vi "Write Roles.vi"(8 "error in (no error)":errorcluster, 10 "Roles":T1, 11 "NormalGamePlay in":refnum<class "NormalGamePlay.lvclass">) -> (0 "error out":errorcluster, 3 "NormalGamePlay out":refnum<class "NormalGamePlay.lvclass">)   [LabVIEW 2020, in "NormalGamePlay.lvclass"]
uses:
  NormalGamePlay.lvclass
  ShootRole_class/ShootRole.lvclass
  FollowAttackerRole_class/FollowAttackerRole.lvclass
  DefaultPsRole_class/DefaultPsRole.lvclass
  NormalGamePlay.lvclass/NormalGamePlay.ctl
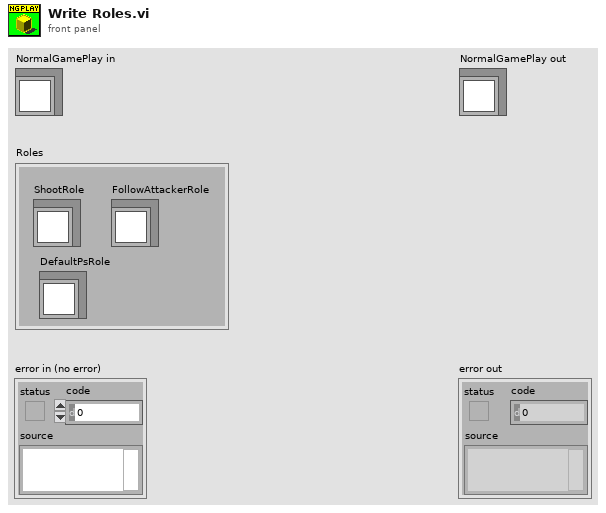
[diagram p1: front panel]
types:
  T1 = cluster{"ShootRole":refnum<class "ShootRole.lvclass">, "FollowAttackerRole":refnum<class "FollowAttackerRole.lvclass">, "DefaultPsRole":refnum<class "DefaultPsRole.lvclass">}
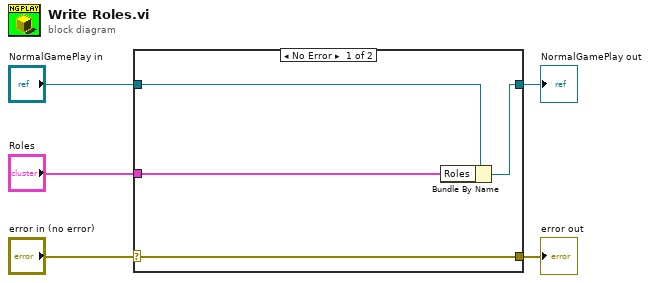
[diagram p0: block diagram]
diagram:
  n1 = case shown="No Error" "error in (no error)" {
    selector: "error in (no error)" -> [w9 w10]
    tunnel: [w9 w10] -> w4
    tunnel: [w7 w11] -> w2
    tunnel: "NormalGamePlay in" -> [w8 w11]
    tunnel: "Roles" -> [w6 _]
    frame No Error {
      n2 = Bundle By Name(cluster=w8, "Roles"=w6) -> (w7:refnum<class "NormalGamePlay.lvclass">)
    }
    frame Error {
    }
  }
  "error out" <- w4
  "NormalGamePlay out" <- w2
